vi "Main packet old.vi"(6 "Enum":enum16{"Disabled", "Teleop"}(ring), 8 "error in (no error)":errorcluster, 11 "SerialPortRef":T1) -> (0 "error out":errorcluster, 3 "SerialPortRef 2":T1)   [LabVIEW 2014]
uses:
  <vilib>/Rock Robotics/WPI/SerialPort/WPI_SerialPortRef.ctl
panel:
  out "String":string
  in  "Battery Voltage":dbl
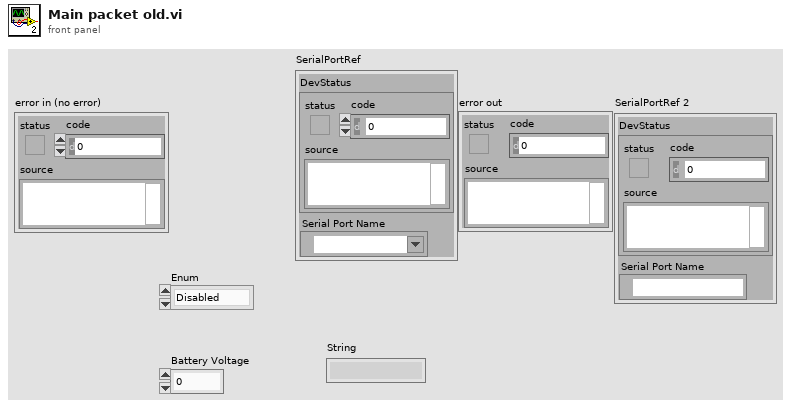
[diagram p1: front panel]
types:
  T1 = typedef "WPI_SerialPortRef.ctl" = cluster{"DevStatus":errorcluster, "Serial Port Name":refnum<visa-resource-name>}
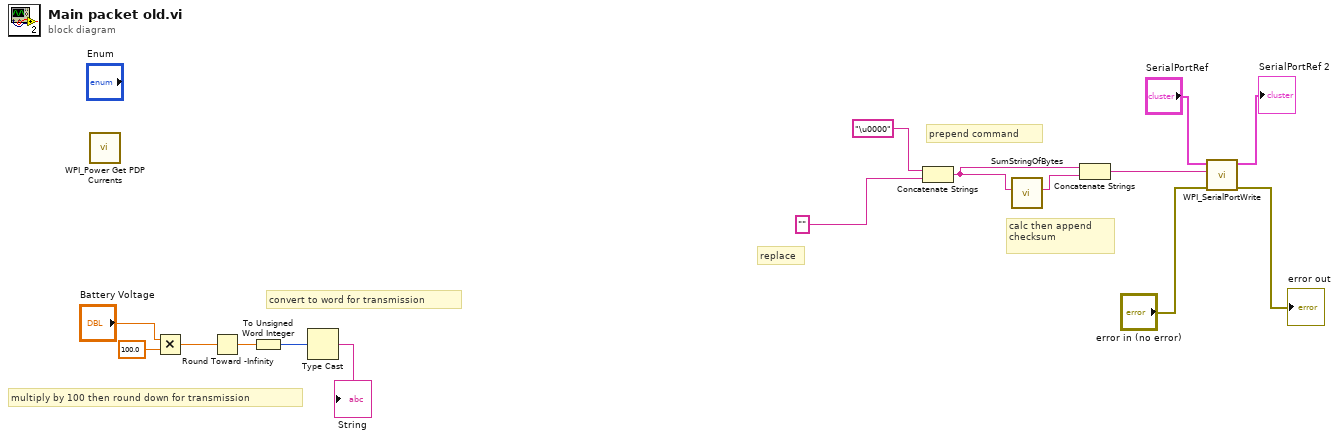
[diagram p0: block diagram]
diagram:
  # "convert to word for transmission"
  # "replace"
  # "calc then append \nchecksum"
  # "prepend command"
  # "multiply by 100 then round down for transmission"
  n1 = call <vilib>:"WPI_Power Get PDP Currents.vi"() -> ()  [unwired: 13 in, 3 out]
  n2 = Multiply(x="Battery Voltage", y=100.0) -> (x*y=w9:dbl)
  n3 = Round Toward -Infinity(1:w9) -> (0:w2:dbl)
  n4 = To Unsigned Word Integer(number=w2) -> (unsigned 16bit integer=w1:u16)
  n5 = Type Cast(x=w1) -> (*(type *) &x=→"String":string)  [unwired: 1 in]
  n6 = Concatenate Strings("\u0000" ("string"), "" ("string")) -> (w6:string)
  n7 = call "SumStringOfBytes.vi"("String Of Bytes"=w6) -> ("SumAsString"=w7:string)  [unwired: 10 in]
  n8 = Concatenate Strings(w6, w7) -> (w8:string)
  n9 = call <vilib>:"WPI_SerialPortWrite.vi"("error in (no error)"="error in (no error)", "Buffer"=w8, "SerialPortRef"="SerialPortRef") -> ("error out"=→"error out":errorcluster, "SerialPortRef"=→"SerialPortRef 2":T1)  [unwired: 6 in, 1 out]
